vi "blink a light.vi"(5 "Whcih Button?":u32, 6 "error in":errorcluster, 7 "Blink Time":dbl, 8 "Button 4":refnum<vi>, 9 "Button 3":refnum<vi>, 10 "Button 2":refnum<vi>, 11 "Button 1":refnum<vi>) -> (4 "error out":errorcluster)   [LabVIEW 2024]
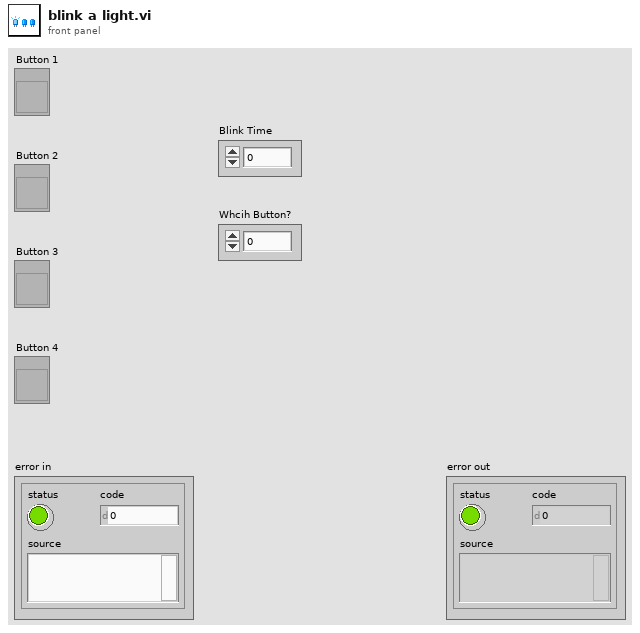
[diagram p1: front panel]
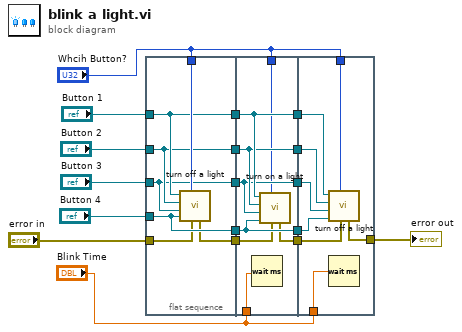
[diagram p0: block diagram]
diagram:
  n1 = flat-sequence {
    tunnel: "Whcih Button?" -> [w25]
    tunnel: "Button 1" -> [w23]
    tunnel: "Button 2" -> [w22]
    tunnel: "Button 3" -> [w21]
    tunnel: "Button 4" -> [w24]
    tunnel: [w24] -> w14
    tunnel: [w23] -> w11
    tunnel: [w22] -> w9
    tunnel: [w21] -> w7
    tunnel: "error in" -> [w20]
    tunnel: [w19] -> w3
    tunnel: "Blink Time" -> [w33]
    tunnel: w14 -> [w32]
    tunnel: [w32] -> w13
    tunnel: [w31] -> w12
    tunnel: w11 -> [w31]
    tunnel: [w30] -> w10
    tunnel: w9 -> [w30]
    tunnel: [w29] -> w8
    tunnel: w7 -> [w29]
    tunnel: "Whcih Button?" -> [w28]
    tunnel: w3 -> [w27]
    tunnel: [w26] -> w2
    tunnel: w13 -> [w41]
    tunnel: w12 -> [w40]
    tunnel: w10 -> [w39]
    tunnel: w8 -> [w38]
    tunnel: "Whcih Button?" -> [w37]
    tunnel: "Blink Time" -> [w36]
    tunnel: w2 -> [w35]
    tunnel: [w34] -> w1
    frame #0 {
      n2 = call "turn off a light.vi"("error in"=w20, "Which Button?"=w25, "Button 4"=w24, "Button 3"=w21, "Button 2"=w22, "Button 1"=w23) -> ("error out"=w19:errorcluster)  [unwired: 5 in]
    }
    frame #1 {
      n3 = Wait (ms)(milliseconds to wait=w33) -> ()  [unwired: 1 out]
      n4 = call "turn on a light.vi"("error in"=w27, "Which Button?"=w28, "Button 4"=w32, "Button 3"=w29, "Button 2"=w30, "Button 1"=w31) -> ("error out"=w26:errorcluster)  [unwired: 5 in]
    }
    frame #2 {
      n5 = call "turn off a light.vi"("error in"=w35, "Which Button?"=w37, "Button 4"=w41, "Button 3"=w38, "Button 2"=w39, "Button 1"=w40) -> ("error out"=w34:errorcluster)  [unwired: 5 in]
      n6 = Wait (ms)(milliseconds to wait=w36) -> ()  [unwired: 1 out]
    }
  }
  "error out" <- w1
